vi "Bind To Type - Empty - Returns Error.vi"() -> ()   [LabVIEW 2017, in "Default Serialization Binder Tests.lvlib"]
uses:
  Default Serialization Binder Tests.lvlib
  Default Serialization Binder/Default Serialization Binder.lvclass
  <vilib>/addons/_JKI Toolkits/Caraya/classes/Assert/Assert Error.vi
  <vilib>/addons/_JKI Toolkits/Caraya/classes/Test/Test.lvclass
  <vilib>/addons/_JKI Toolkits/Caraya/classes/Assert/Assert.lvclass
panel:
  out "error out":errorcluster
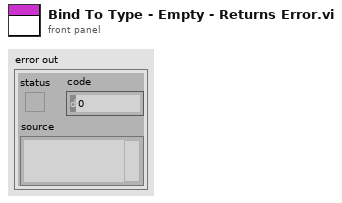
[diagram p1: front panel]
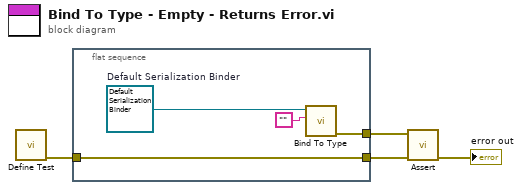
[diagram p0: block diagram]
diagram:
  n1 = call <vilib>:"Define Test.vi"() -> ("error out"=w1:errorcluster)  [unwired: 11 in]
  n2 = flat-sequence {
    tunnel: [w6] -> w3
    tunnel: [w5] -> w2
    tunnel: w1 -> [w5]
    frame #0 {
      w8 = refnum<class "Default Serialization Binder.lvclass"> refnum  # Default Serialization Binder
      n3 = call-dynamic "Bind To Type.vi"("Type Name"="", "Default Serialization Binder in"=w8) -> ("error out"=w6:errorcluster)  [unwired: 7 in, 2 out]
    }
  }
  n4 = call-poly <vilib>:"Assert.vi"("error in (no error)"=w2, "Error?"=w3) -> ("error out"=→"error out":errorcluster)  [unwired: 9 in]
